vi "GenFunc.vi"(0 "amplitude":dbl=1.0 format="%0.2p", 1 "offset":dbl format="%0.2p", 5 "frequency":dbl=10.0 format="%0.2p", 7 "noiseRMS":dbl=1.0 format="%.2p", 9 "signal type":T1(ring), 11 "error in (no error)":errorcluster, 12 "sampling info":cluster{"Fs":dbl, "#s":dbl}={"Fs"=1000.0, "#s"=1000.0} {"Fs" format="%.2p"}) -> (6 "signal out":waveform(dbl)(graph), 15 "error out":errorcluster)   [LabVIEW 2025]
uses:
  <vilib>/measure/NI_MABase.lvlib
panel:
  # "Un generador de funciones. Puedes generar una onda y añadirle ruido (noiseRMS)"
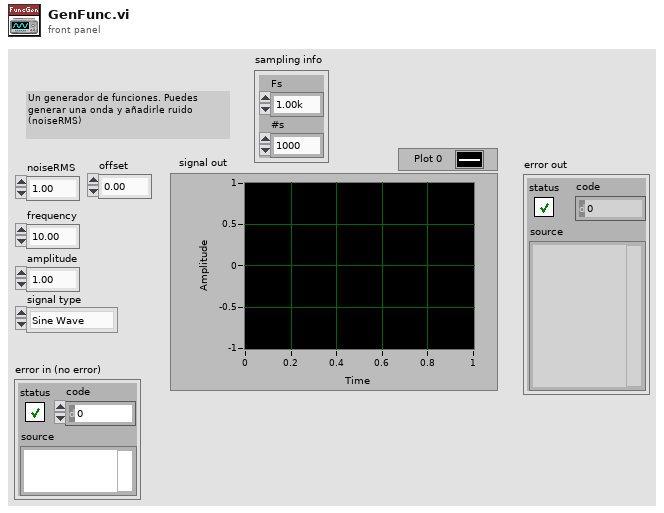
[diagram p1: front panel]
types:
  T1 = enum16{"Sine Wave", "Triangle Wave", "Square Wave", "Sawtooth Wave"}
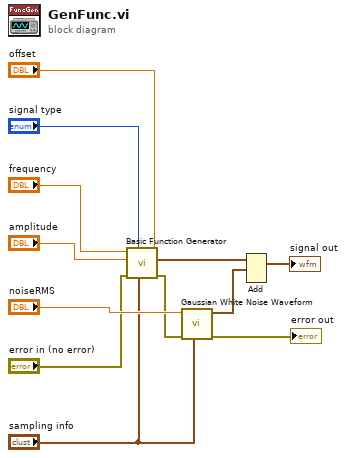
[diagram p0: block diagram]
diagram:
  n1 = call <vilib>:"Basic Function Generator.vi"("offset"="offset", "sampling info"="sampling info", "signal type"="signal type", "error in (no error)"="error in (no error)", "amplitude"="amplitude", "frequency"="frequency") -> ("error out"=w5:errorcluster, "signal out"=w8:waveform(dbl))  [unwired: 3 in, 1 out]
  n2 = call <vilib>:"Gaussian White Noise Waveform.vi"("sampling info"="sampling info", "error in (no error)"=w5, "standard deviation"="noiseRMS") -> ("error out"=→"error out":errorcluster, "signal out"=w7:waveform(dbl))  [unwired: 7 in]
  n3 = Add(1:w7, 2:w8) -> (0:→"signal out":waveform(dbl))  [unwired: 1 in, 1 out]
